vi "Generate Waveform (Multi-Array).vi"(0 "number of samples":u32=300000 caption="Number of Samples", 5 "sample rate":dbl=10000000.0 caption="Sample Rate" format="%#.3pS/s", 11 "x":cdb[](array[numeric])) -> (4 "I":i16[](array[numeric]), 6 "Q":i16[](array[numeric]), 15 "error out":errorcluster)   [LabVIEW 2015]
doc: "Creates a waveform to send to a device for generation.\n\n<B>Input Parameters</B>\n\n<B>number of samples</B> in the generated waveform.\n\n<B>sample rate</B> is the rate, in samples per second, that will be used to create the waveform.\n\n<B>tone frequency</B> is the frequency of the tone, in hertz, to generate.\n\n<B>amplitude</B> is used to set the amplitude of the tone. DSP overflow will occur if the 'amplitude' is too high.\n\n<B>Output Parameters</B>\n\n<B>I</B> is the real (I) portion of the generated waveform.\n\n<B>Q</B> is the imaginary (Q) portion of the generated waveform.\n\n<B>Waveform</B> is the generated waveform.\n\n<B>error out</B> contains error information. This output provides standard 'error out' functionality."
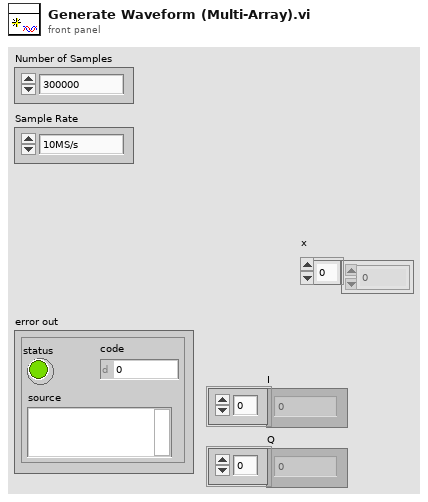
[diagram p1: front panel]
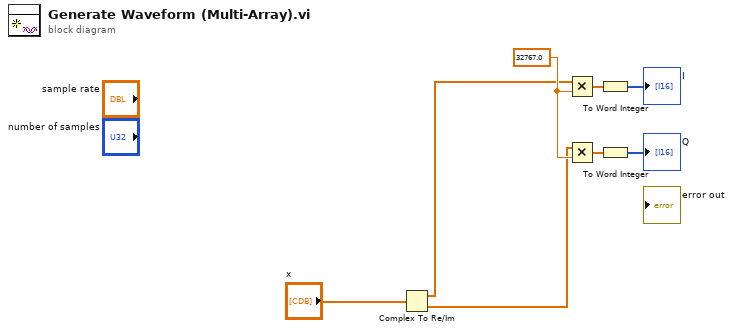
[diagram p0: block diagram]
diagram:
  w6 = 32767.0
  n1 = Complex To Re/Im(x + iy="x") -> (x=w4:dbl[], y=w3:dbl[])
  n2 = Multiply(x=w4, y=w6) -> (x*y=w7:dbl[])
  n3 = Multiply(x=w3, y=w6) -> (x*y=w8:dbl[])
  n4 = To Word Integer(number=w7) -> (16bit integer=→"I":i16[])
  n5 = To Word Integer(number=w8) -> (16bit integer=→"Q":i16[])
